vi "KH_DAQ_TURCK_FGlob_AO_Status.vi"(5 "Function (Recall One)":T1=enum."Recall one", 8 "err in":errorcluster caption="error", 10 "AO Status IN":bool[](array[boolean])) -> (0 "err out":errorcluster caption="error", 2 "AO Status OUT":bool[](array[boolean]))   [LabVIEW 2021]
uses:
  KH Turck EthernetIP 17.12/KH TURCK TypeDefs FGlob.ctl
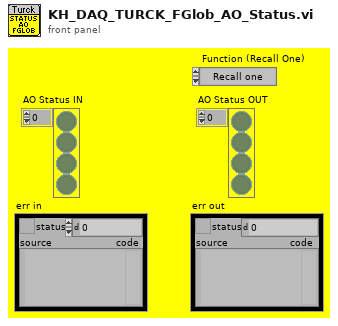
[diagram p1: front panel]
types:
  T1 = typedef "KH TURCK TypeDefs FGlob.ctl" = enum16{"Put one", "Put all", "Recall one", "Recall all"}
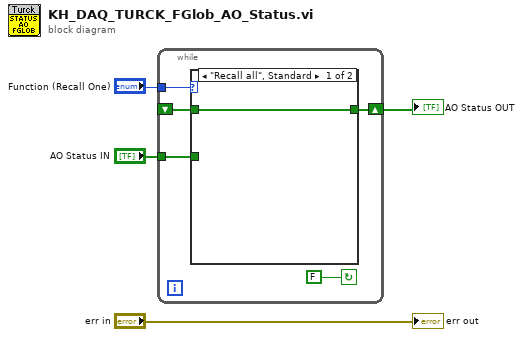
[diagram p0: block diagram]
diagram:
  n1 = while {
    shift-right: [w7] -> w2
    shift-left: _ -> [w6]
    tunnel: "Function (Recall One)" -> [w8]
    tunnel: "AO Status IN" -> [w5]
    stop <- FALSE continue-if-true
    n2 = case shown="\"Recall all\", Standard" w8 {
      tunnel: [w10 w11] -> w7
      tunnel: w6 -> [w10 _]
      tunnel: w5 -> [_ w11]
      frame "Recall all", Default {
      }
      frame "Put all" {
      }
    }
  }
  "AO Status OUT" <- w2
  "err out" <- "err in"
